vi "SOL Instruments MS.vi"() -> ()   [LabVIEW 2015]
doc: "Example VI that demonstrates all library features."
uses:
  PL SOL Instruments MS.lvclass
panel:
  in  "slit configuration":cluster{"width, um":dbl, "reset":bool}
  in  "slit":u8(ring)
  in  "mirror position index":u8(ring)
  in  "mirror":u8(ring)
  in  "shutter state":bool
  in  "shutter":u8(ring) items=["Shutter S1"]
  in  "turret configuration":T1 {"grating" items=["1200; 750", "1200; 280"]}
  in  "turret":u8(ring) items=["Change of the gratings"]
  in  "configuration file path":path
  out "SOL MS":refnum<class "PL SOL Instruments MS.lvclass">
  in  "port":refnum<visa-resource-name>
  out "error":errorcluster
  in  "stop":bool
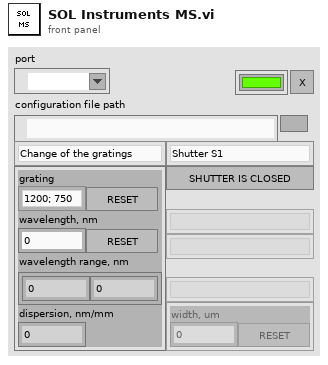
[diagram p1: front panel]
types:
  T1 = cluster{"grating":u8, "reset grating":bool, "wavelength, nm":dbl, "reset wavelength":bool, "wavelength range, nm":cluster{"min":dbl, "max":dbl}, "dispersion, nm/mm":dbl}
  T2 = cluster{"turrets":cluster{"name":string, "gratings":cluster{"name":string, "groove density, g/mm":dbl, "blaze wavelength, nm":dbl, "min wavelength, nm":dbl, "max wavelength, nm":dbl}[]}[], "shutters":cluster{"name":string}[], "mirrors":cluster{"name":string, "positions":cluster{"name":string}[]}[], "slits":cluster{"name":string, "min width, um":dbl, "max width, um":dbl}[]}
  T3 = cluster{"turrets":cluster{"current grating index":u8, "wavelength, nm":dbl, "dispersion, nm/mm":dbl}[], "shutters":cluster{"is open":bool}[], "mirrors":cluster{"current position index":u8}[], "slits":cluster{"width, um":dbl}[]}
  T4 = cluster{"name":string, "gratings":cluster{"name":string, "groove density, g/mm":dbl, "blaze wavelength, nm":dbl, "min wavelength, nm":dbl, "max wavelength, nm":dbl}[]}[]
  T5 = cluster{"current grating index":u8, "wavelength, nm":dbl, "dispersion, nm/mm":dbl}[]
  T6 = cluster{"name":string, "gratings":cluster{"name":string, "groove density, g/mm":dbl, "blaze wavelength, nm":dbl, "min wavelength, nm":dbl, "max wavelength, nm":dbl}[]}
  T7 = cluster{"current grating index":u8, "wavelength, nm":dbl, "dispersion, nm/mm":dbl}
  T8 = cluster{"name":string, "groove density, g/mm":dbl, "blaze wavelength, nm":dbl, "min wavelength, nm":dbl, "max wavelength, nm":dbl}[]
  T9 = cluster{"name":string, "groove density, g/mm":dbl, "blaze wavelength, nm":dbl, "min wavelength, nm":dbl, "max wavelength, nm":dbl}
  T10 = cluster{"name":string, "positions":cluster{"name":string}[]}[]
  T11 = cluster{"name":string, "positions":cluster{"name":string}[]}
  T12 = enum8{"Enabled", "Disabled", "Disabled and Grayed Out"}
  T13 = cluster{"name":string, "min width, um":dbl, "max width, um":dbl}[]
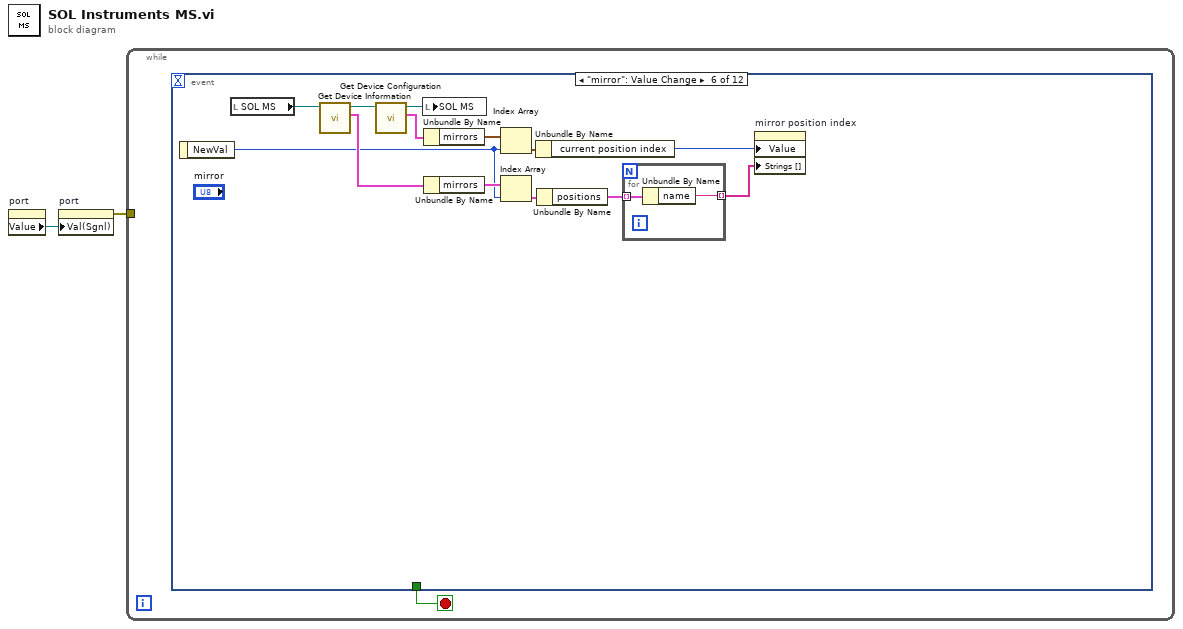
[diagram p0: block diagram]
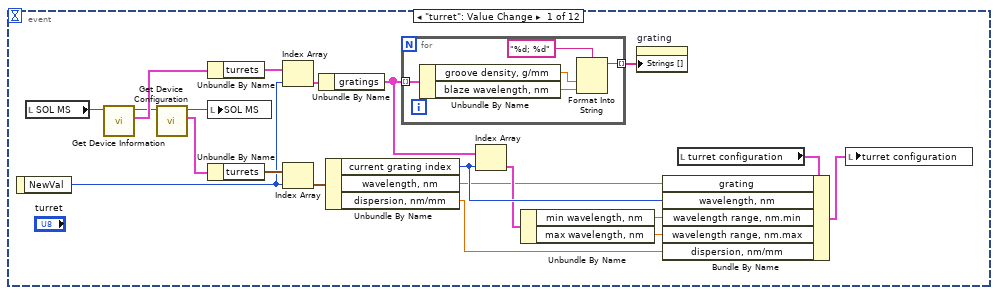
[diagram p2: hidden frame]
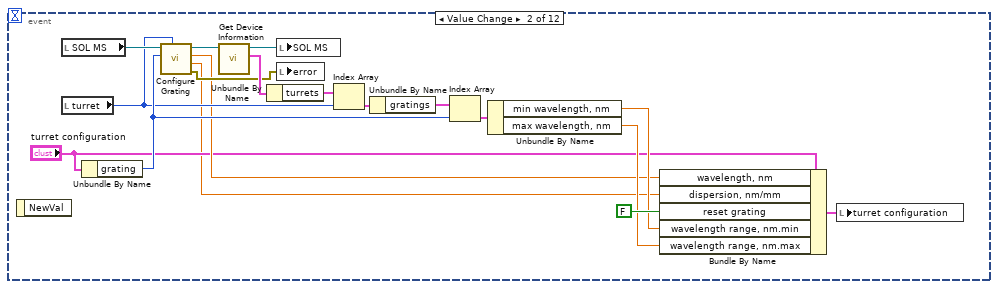
[diagram p3: hidden frame]
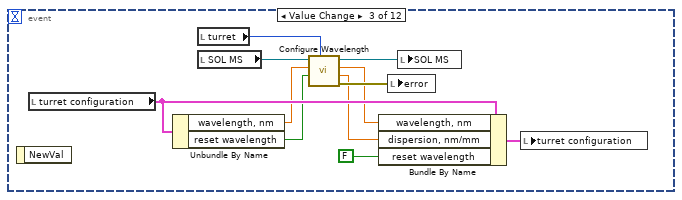
[diagram p4: hidden frame]
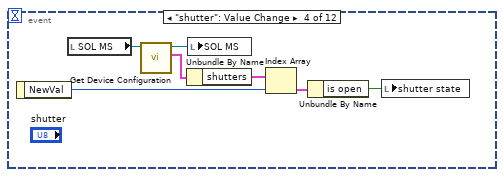
[diagram p5: hidden frame]
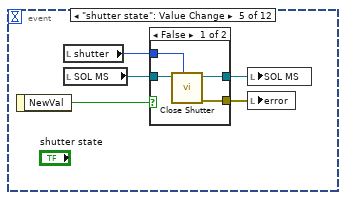
[diagram p6: hidden frame]
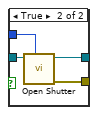
[diagram p7: hidden frame]
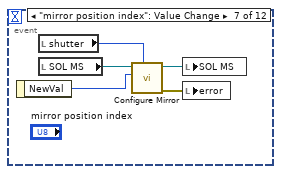
[diagram p8: hidden frame]
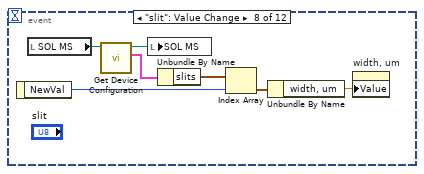
[diagram p9: hidden frame]
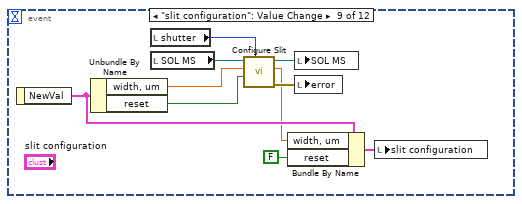
[diagram p10: hidden frame]
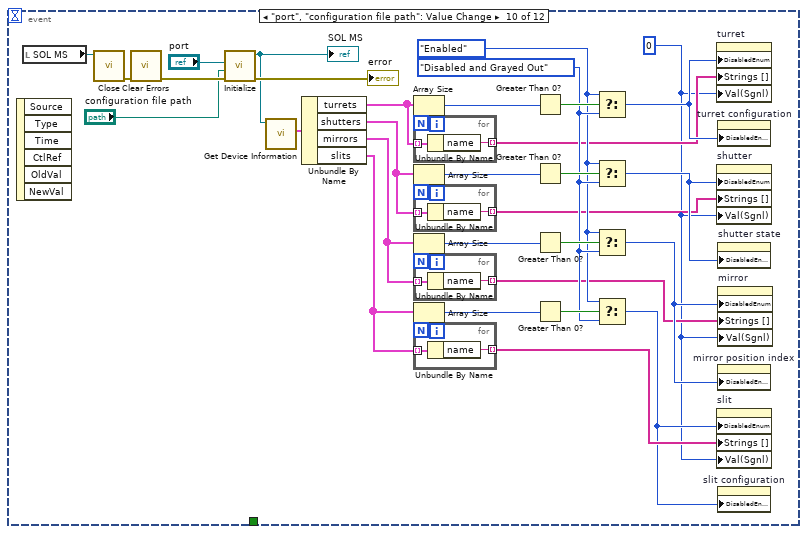
[diagram p11: hidden frame]
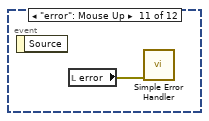
[diagram p12: hidden frame]
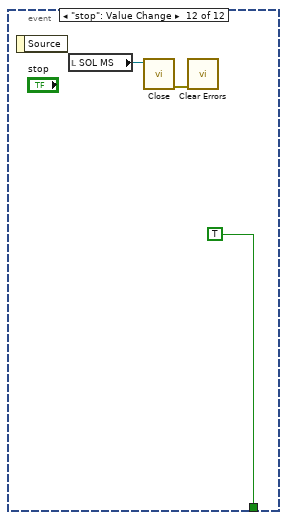
[diagram p13: hidden frame]
diagram:
  n1 = property on="port" class="VISAName"() -> ("Value"=w1:refnum<visa-resource-name>)  [unwired: 2 in, 2 out]
  n2 = property on="port" class="VISAName"("Val(Sgnl)"=w1) -> (error out=w2:errorcluster)  [unwired: 2 in, 1 out]
  n3 = while {
    tunnel: w2 -> [_]
    stop <- w3 stop-if-true
    n4 = event shown="[5] \"mirror\": Value Change" {
      selector: _ -> [_ _ _ _ _ _ _ _ _ _ _ _]
      dyn-events: _ -> [_ _ _ _ _ _ _ _ _ _ _ _]
      timeout: _ -> [_ _ _ _ _ _ _ _ _ _ _ _]
      tunnel: [_ _ _ _ _ _ _ _ _ _ _ TRUE ("stop")] -> w3
      event "turret": Value Change {
        n5 = event-data() -> ("NewVal"=w9:u8)  [unwired: 1 in]
        n6 = local read "SOL MS"() -> (w8:refnum<class "PL SOL Instruments MS.lvclass">)
        n7 = call "Get Device Information.vi"("SOL MS in"=w8) -> ("info"=w7:T2, "SOL MS out"=w6:refnum<class "PL SOL Instruments MS.lvclass">)  [unwired: 9 in]
        n8 = call "Get Device Configuration.vi"("SOL MS in"=w6) -> ("configuration"=w4:T3, "SOL MS out"=w5:refnum<class "PL SOL Instruments MS.lvclass">)  [unwired: 9 in]
        n9 = Unbundle By Name(w7) -> ("turrets"=w22:T4)
        n10 = local write "SOL MS"(w5) -> ()
        n11 = Unbundle By Name(w4) -> ("turrets"=w23:T5)
        n12 = Index Array(array=w22, index=w9) -> (element=w20:T6)
        n13 = Index Array(array=w23, index=w9) -> (element=w21:T7)
        n14 = Unbundle By Name(w20) -> ("gratings"=w16:T8)
        n15 = Unbundle By Name(w21) -> ("current grating index"=w15:u8, "wavelength, nm"=w13:dbl, "dispersion, nm/mm"=w10:dbl)
        n16 = for {
          tunnel: w16 -> [w28] mode=indexing
          tunnel: [w24] -> w17 mode=indexing
          n17 = Unbundle By Name(w28) -> ("groove density, g/mm"=w26:dbl, "blaze wavelength, nm"=w25:dbl)
          n18 = Format Into String(format string="%d; %d", w26, w25) -> (resulting string=w24:string)  [unwired: 2 in, 1 out]
        }
        n19 = Index Array(array=w16, index=w15) -> (element=w14:T9)
        n20 = Unbundle By Name(w14) -> ("min wavelength, nm"=w12:dbl, "max wavelength, nm"=w11:dbl)
        n21 = property on="grating" class="Ring (strict)"("Strings []"=w17) -> ()  [unwired: 2 in, 2 out]
        n22 = local read "turret configuration"() -> (w19:T1)
        n23 = Bundle By Name(cluster=w19, "grating"=w13, "wavelength, nm"=w15, "wavelength range, nm.min"=w12, "wavelength range, nm.max"=w11, "dispersion, nm/mm"=w10) -> (w18:T1)
        n24 = local write "turret configuration"(w18) -> ()
      }
      event "turret configuration.grating", "turret configuration.reset grating": Value Change {
        n25 = event-data() -> ()  [unwired: 1 in, 1 out]
        n26 = local read "SOL MS"() -> (w39:refnum<class "PL SOL Instruments MS.lvclass">)
        n27 = local read "turret"() -> (w37:u8)
        n28 = Unbundle By Name("turret configuration") -> ("grating"=w38:u8)
        n29 = call "Configure Grating.vi"("turret index (0)"=w37, "grating index"=w38, "SOL MS in"=w39) -> ("error out"=w33:errorcluster, "dispersion, nm/mm"=w30:dbl, "wavelength, nm"=w32:dbl, "SOL MS out"=w35:refnum<class "PL SOL Instruments MS.lvclass">)  [unwired: 5 in]
        n30 = call "Get Device Information.vi"("SOL MS in"=w35) -> ("info"=w34:T2, "SOL MS out"=w36:refnum<class "PL SOL Instruments MS.lvclass">)  [unwired: 9 in]
        n31 = Unbundle By Name(w34) -> ("turrets"=w45:T4)
        n32 = local write "SOL MS"(w36) -> ()
        n33 = local write "error"(w33) -> ()
        n34 = Index Array(array=w45, index=w37) -> (element=w44:T6)
        n35 = Unbundle By Name(w44) -> ("gratings"=w43:T8)
        n36 = Index Array(array=w43, index=w38) -> (element=w42:T9)
        n37 = Unbundle By Name(w42) -> ("min wavelength, nm"=w41:dbl, "max wavelength, nm"=w40:dbl)
        n38 = Bundle By Name(cluster="turret configuration", "wavelength, nm"=w32, "dispersion, nm/mm"=w30, "reset grating"=FALSE ("reset wavelength"), "wavelength range, nm.min"=w41, "wavelength range, nm.max"=w40) -> (w29:T1)
        n39 = local write "turret configuration"(w29) -> ()
      }
      event "turret configuration.wavelength, nm", "turret configuration.reset wavelength": Value Change {
        n40 = event-data() -> ()  [unwired: 1 in, 1 out]
        n41 = local read "turret configuration"() -> (w56:T1)
        n42 = Unbundle By Name(w56) -> ("wavelength, nm"=w52:dbl, "reset wavelength"=w51:bool)
        n43 = local read "turret"() -> (w53:u8)
        n44 = local read "SOL MS"() -> (w54:refnum<class "PL SOL Instruments MS.lvclass">)
        n45 = call "Configure Wavelength.vi"("turret index (0)"=w53, "reset (false)"=w51, "wavelength, nm"=w52, "SOL MS in"=w54) -> ("error out"=w50:errorcluster, "dispersion, nm/mm"=w47:dbl, "wavelength, nm"=w48:dbl, "SOL MS out"=w49:refnum<class "PL SOL Instruments MS.lvclass">)  [unwired: 4 in]
        n46 = Bundle By Name(cluster=w56, "wavelength, nm"=w48, "dispersion, nm/mm"=w47, "reset wavelength"=FALSE) -> (w55:T1)
        n47 = local write "error"(w50) -> ()
        n48 = local write "SOL MS"(w49) -> ()
        n49 = local write "turret configuration"(w55) -> ()
      }
      event "shutter": Value Change {
        n50 = event-data() -> ("NewVal"=w61:u8)  [unwired: 1 in]
        n51 = local read "SOL MS"() -> (w60:refnum<class "PL SOL Instruments MS.lvclass">)
        n52 = call "Get Device Configuration.vi"("SOL MS in"=w60) -> ("configuration"=w58:T3, "SOL MS out"=w59:refnum<class "PL SOL Instruments MS.lvclass">)  [unwired: 9 in]
        n53 = Unbundle By Name(w58) -> ("shutters"=w64:cluster{"is open":bool}[])
        n54 = local write "SOL MS"(w59) -> ()
        n55 = Index Array(array=w64, index=w61) -> (element=w63:cluster{"is open":bool})
        n56 = Unbundle By Name(w63) -> ("is open"=w62:bool)
        n57 = local write "shutter state"(w62) -> ()
      }
      event "shutter state": Value Change {
        n58 = event-data() -> ("NewVal"=w69:bool)  [unwired: 1 in]
        n59 = local read "shutter"() -> (w67:u8)
        n60 = local read "SOL MS"() -> (w68:refnum<class "PL SOL Instruments MS.lvclass">)
        n61 = case shown="False" w69 {
          tunnel: w68 -> [w73 w77]
          tunnel: w67 -> [w70 w76]
          tunnel: [w72 w75] -> w66
          tunnel: [w71 w74] -> w65
          frame False {
            n62 = call "Close Shutter.vi"("shutter index (0)"=w70, "SOL MS in"=w73) -> ("error out"=w71:errorcluster, "SOL MS out"=w72:refnum<class "PL SOL Instruments MS.lvclass">)  [unwired: 8 in]
          }
          frame True {
            n63 = call "Open Shutter.vi"("shutter index (0)"=w76, "SOL MS in"=w77) -> ("error out"=w74:errorcluster, "SOL MS out"=w75:refnum<class "PL SOL Instruments MS.lvclass">)  [unwired: 8 in]
          }
        }
        n64 = local write "SOL MS"(w66) -> ()
        n65 = local write "error"(w65) -> ()
      }
      event "mirror": Value Change {
        n66 = event-data() -> ("NewVal"=w82:u8)  [unwired: 1 in]
        n67 = local read "SOL MS"() -> (w86:refnum<class "PL SOL Instruments MS.lvclass">)
        n68 = call "Get Device Information.vi"("SOL MS in"=w86) -> ("info"=w84:T2, "SOL MS out"=w85:refnum<class "PL SOL Instruments MS.lvclass">)  [unwired: 9 in]
        n69 = call "Get Device Configuration.vi"("SOL MS in"=w85) -> ("configuration"=w87:T3, "SOL MS out"=w88:refnum<class "PL SOL Instruments MS.lvclass">)  [unwired: 9 in]
        n70 = local write "SOL MS"(w88) -> ()
        n71 = Unbundle By Name(w87) -> ("mirrors"=w90:cluster{"current position index":u8}[])
        n72 = Unbundle By Name(w84) -> ("mirrors"=w83:T10)
        n73 = Index Array(array=w90, index=w82) -> (element=w89:cluster{"current position index":u8})
        n74 = Index Array(array=w83, index=w82) -> (element=w81:T11)
        n75 = Unbundle By Name(w89) -> ("current position index"=w80:u8)
        n76 = Unbundle By Name(w81) -> ("positions"=w79:cluster{"name":string}[])
        n77 = for {
          tunnel: w79 -> [w92] mode=indexing
          tunnel: [w91] -> w78 mode=indexing
          n78 = Unbundle By Name(w92) -> ("name"=w91:string)
        }
        n79 = property on="mirror position index" class="Ring (strict)"("Value"=w80, "Strings []"=w78) -> ()  [unwired: 2 in, 2 out]
      }
      event "mirror position index": Value Change {
        n80 = event-data() -> ("NewVal"=w93:u8)  [unwired: 1 in]
        n81 = local read "shutter"() -> (w94:u8)
        n82 = local read "SOL MS"() -> (w97:refnum<class "PL SOL Instruments MS.lvclass">)
        n83 = call "Configure Mirror.vi"("mirror index (0)"=w94, "mirror position index"=w93, "SOL MS in"=w97) -> ("error out"=w95:errorcluster, "SOL MS out"=w96:refnum<class "PL SOL Instruments MS.lvclass">)  [unwired: 7 in]
        n84 = local write "SOL MS"(w96) -> ()
        n85 = local write "error"(w95) -> ()
      }
      event "slit": Value Change {
        n86 = event-data() -> ("NewVal"=w102:u8)  [unwired: 1 in]
        n87 = local read "SOL MS"() -> (w101:refnum<class "PL SOL Instruments MS.lvclass">)
        n88 = call "Get Device Configuration.vi"("SOL MS in"=w101) -> ("configuration"=w99:T3, "SOL MS out"=w100:refnum<class "PL SOL Instruments MS.lvclass">)  [unwired: 9 in]
        n89 = local write "SOL MS"(w100) -> ()
        n90 = Unbundle By Name(w99) -> ("slits"=w104:cluster{"width, um":dbl}[])
        n91 = Index Array(array=w104, index=w102) -> (element=w103:cluster{"width, um":dbl})
        n92 = Unbundle By Name(w103) -> ("width, um"=w98:dbl)
        n93 = property on="width, um" class="DigNum (strict)"("Value"=w98) -> ()  [unwired: 2 in, 2 out]
      }
      event "slit configuration": Value Change {
        n94 = event-data() -> ("NewVal"=w108:cluster{"width, um":dbl, "reset":bool})  [unwired: 1 in]
        n95 = Unbundle By Name(w108) -> ("width, um"=w110:dbl, "reset"=w109:bool)
        n96 = local read "shutter"() -> (w114:u8)
        n97 = local read "SOL MS"() -> (w111:refnum<class "PL SOL Instruments MS.lvclass">)
        n98 = call "Configure Slit.vi"("slit index (0)"=w114, "reset (false)"=w109, "width, um"=w110, "SOL MS in"=w111) -> ("error out"=w112:errorcluster, "width, um"=w106:dbl, "SOL MS out"=w113:refnum<class "PL SOL Instruments MS.lvclass">)  [unwired: 5 in]
        n99 = Bundle By Name(cluster=w108, "width, um"=w106, "reset"=FALSE) -> (w107:cluster{"width, um":dbl, "reset":bool})
        n100 = local write "SOL MS"(w113) -> ()
        n101 = local write "error"(w112) -> ()
        n102 = local write "slit configuration"(w107) -> ()
      }
      event "port", "configuration file path": Value Change {
        w115 = u8 0 ("Value (Signaling)")
        w125 = T12."Disabled and Grayed Out" ("Disabled")
        w124 = T12."Enabled" ("Disabled")
        n103 = event-data() -> ()  [unwired: 1 in, 6 out]
        n104 = local read "SOL MS"() -> (w145:refnum<class "PL SOL Instruments MS.lvclass">)
        n105 = call "Close.vi"("SOL MS in"=w145) -> ("error out"=w143:errorcluster)  [unwired: 10 in]
        n106 = call <vilib>:"Clear Errors.vi"("error in (no error)"=w143) -> ("error out"=w144:errorcluster)  [unwired: 5 in, 1 out]
        n107 = call "Initialize.vi"("error in (no error)"=w144, "configuration file path"="configuration file path", "port"="port") -> ("error out"=→"error":errorcluster, "SOL MS out"=w139:refnum<class "PL SOL Instruments MS.lvclass">)  [unwired: 7 in]
        "SOL MS" <- w139
        n108 = call "Get Device Information.vi"("SOL MS in"=w139) -> ("info"=w138:T2)  [unwired: 9 in, 1 out]
        n109 = Unbundle By Name(w138) -> ("turrets"=w134:T4, "shutters"=w135:cluster{"name":string}[], "mirrors"=w136:T10, "slits"=w137:T13)
        n110 = Array Size(array=w134) -> (size(s)=w133:i32)
        n111 = for {
          tunnel: w134 -> [w153] mode=indexing
          tunnel: [w152] -> w122 mode=indexing
          n112 = Unbundle By Name(w153) -> ("name"=w152:string)
        }
        n113 = Array Size(array=w135) -> (size(s)=w131:i32)
        n114 = for {
          tunnel: w135 -> [w151] mode=indexing
          tunnel: [w150] -> w120 mode=indexing
          n115 = Unbundle By Name(w151) -> ("name"=w150:string)
        }
        n116 = Array Size(array=w136) -> (size(s)=w129:i32)
        n117 = for {
          tunnel: w136 -> [w149] mode=indexing
          tunnel: [w148] -> w118 mode=indexing
          n118 = Unbundle By Name(w149) -> ("name"=w148:string)
        }
        n119 = Array Size(array=w137) -> (size(s)=w126:i32)
        n120 = for {
          tunnel: w137 -> [w147] mode=indexing
          tunnel: [w146] -> w117 mode=indexing
          n121 = Unbundle By Name(w147) -> ("name"=w146:string)
        }
        n122 = Greater Than 0?(x=w133) -> (x > 0?=w132:bool)
        n123 = Greater Than 0?(x=w131) -> (x > 0?=w130:bool)
        n124 = Greater Than 0?(x=w129) -> (x > 0?=w128:bool)
        n125 = Greater Than 0?(x=w126) -> (x > 0?=w127:bool)
        n126 = Select(t=w124, s=w132, f=w125) -> (s? t:f=w123:T12)
        n127 = Select(t=w124, s=w130, f=w125) -> (s? t:f=w121:T12)
        n128 = Select(t=w124, s=w128, f=w125) -> (s? t:f=w119:T12)
        n129 = Select(t=w124, s=w127, f=w125) -> (s? t:f=w116:T12)
        n130 = property on="turret" class="Ring (strict)"("DisabledEnum"=w123, "Strings []"=w122, "Val(Sgnl)"=w115) -> ()  [unwired: 2 in, 2 out]
        n131 = property on="shutter" class="Ring (strict)"("DisabledEnum"=w121, "Strings []"=w120, "Val(Sgnl)"=w115) -> ()  [unwired: 2 in, 2 out]
        n132 = property on="slit" class="Ring (strict)"("DisabledEnum"=w116, "Strings []"=w117, "Val(Sgnl)"=w115) -> ()  [unwired: 2 in, 2 out]
        n133 = property on="turret configuration" class="Clust (strict)"("DisabledEnum"=w123) -> ()  [unwired: 2 in, 2 out]
        n134 = property on="shutter state" class="Bool (strict)"("DisabledEnum"=w121) -> ()  [unwired: 2 in, 2 out]
        n135 = property on="mirror" class="Ring (strict)"("DisabledEnum"=w119, "Strings []"=w118, "Val(Sgnl)"=w115) -> ()  [unwired: 2 in, 2 out]
        n136 = property on="mirror position index" class="Ring (strict)"("DisabledEnum"=w119) -> ()  [unwired: 2 in, 2 out]
        n137 = property on="slit configuration" class="Clust (strict)"("DisabledEnum"=w116) -> ()  [unwired: 2 in, 2 out]
      }
      event "error": Mouse Up {
        n138 = event-data() -> ()  [unwired: 1 in, 1 out]
        n139 = local read "error"() -> (w154:errorcluster)
        n140 = call <vilib>:"Simple Error Handler.vi"("error in (no error)"=w154) -> ()  [unwired: 4 in, 5 out]
      }
      event "stop": Value Change {
        n141 = event-data() -> ()  [unwired: 1 in, 1 out]
        n142 = local read "SOL MS"() -> (w156:refnum<class "PL SOL Instruments MS.lvclass">)
        n143 = call "Close.vi"("SOL MS in"=w156) -> ("error out"=w155:errorcluster)  [unwired: 10 in]
        n144 = call <vilib>:"Clear Errors.vi"("error in (no error)"=w155) -> ()  [unwired: 5 in, 2 out]
      }
    }
  }
